vi "资讯打标签-打印函数 - 副本.vi"(6 "错误输入（无错误）":errorcluster caption="print error in", 7 "label num":i32, 8 "print path local":bool, 9 "PRINT":refnum<k24>, 10 "SN":refnum<k24>, 11 "SN输入":string="000019120-SD-R/Z00A2R1553S") -> (3 "printPath":string, 4 "print error":errorcluster caption="print error out")   [LabVIEW 2011]
uses:
  Data/ClassLibraryMisWebservice.dll
panel:
  out "Temp":string
  out "strPrintContent":string
  out "PrintSFCFSNLabel":string="OK"
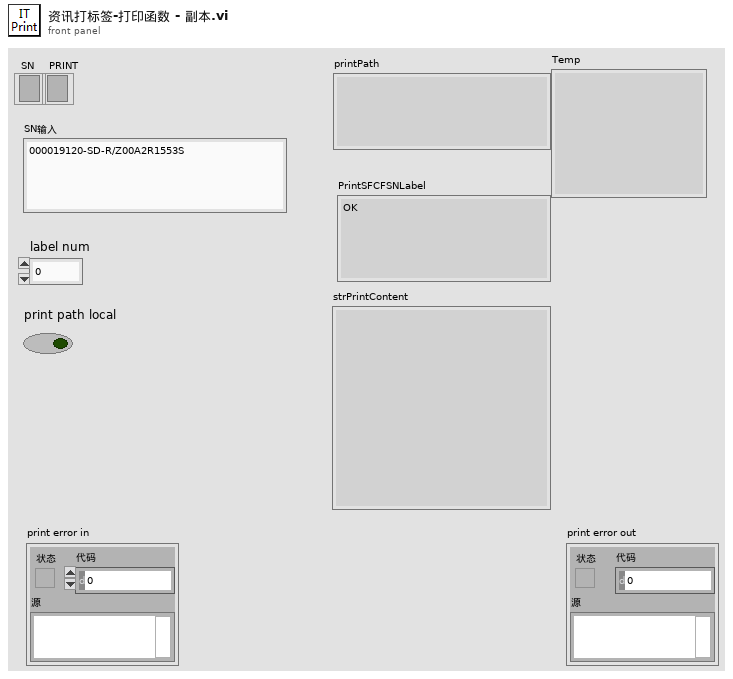
[diagram p1: front panel]
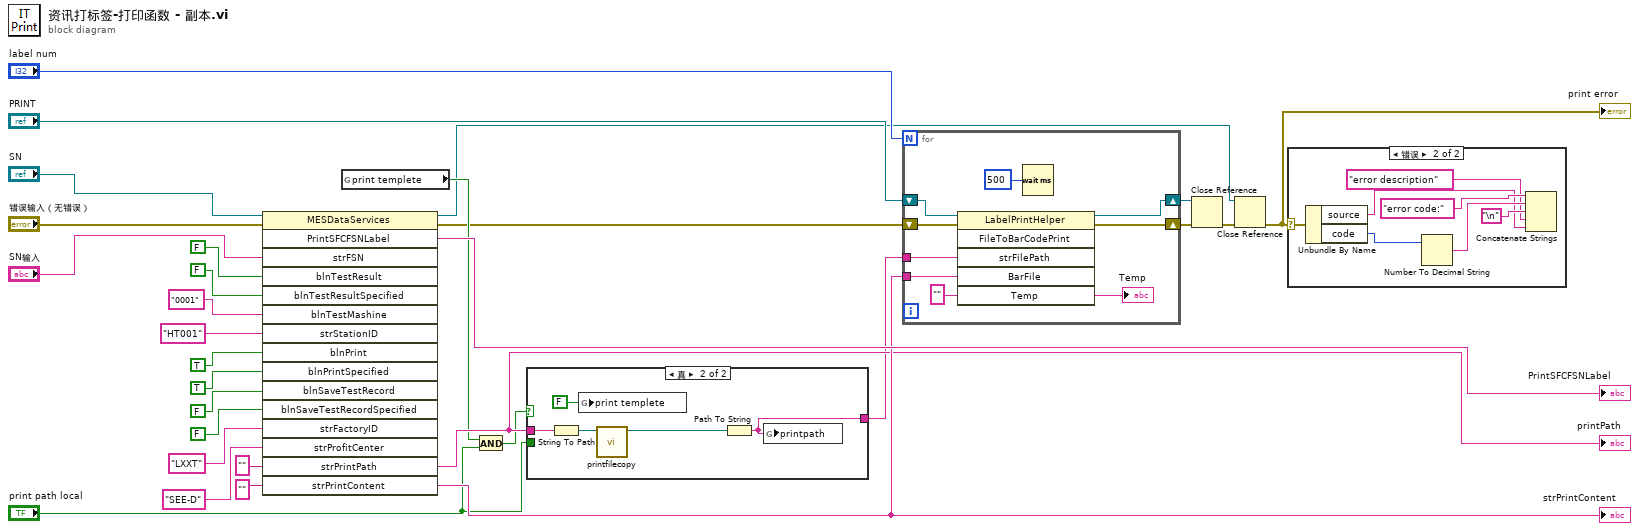
[diagram p0: block diagram]
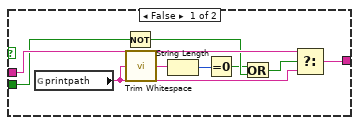
[diagram p3: hidden frame]
diagram:
  n1 = invoke class="MESDataServices" method="PrintSFCFSNLabel"(reference="SN", error in="错误输入（无错误）", "strFSN"="SN输入", "blnTestResult"=FALSE, "blnTestResultSpecified"=FALSE, "blnTestMashine"="0001", "strStationID"="HT001", "blnPrint"=TRUE, "blnPrintSpecified"=TRUE, "blnSaveTestRecord"=FALSE, "blnSaveTestRecordSpecified"=FALSE, "strFactoryID"="LXXT", "strProfitCenter"="SEE-D", "strPrintPath"="" ("printPath"), "strPrintContent"="") -> (reference out=w2:refnum<k24>, error out=w8:errorcluster, "PrintSFCFSNLabel"=→"PrintSFCFSNLabel":string, "strPrintPath"=w14:string, "strPrintContent"=w16:string)  [unwired: 1 in, 11 out]
  "printPath" <- w14
  "strPrintContent" <- w16
  n2 = global read "全局.vi" "print templete"() -> (w12:bool)
  n3 = And(x=w12, y="print path local") -> (x .and. y?=w11:bool)
  n4 = case shown="真" w11 {
    tunnel: w14 -> [w37 w44]
    tunnel: [w35 w40] -> w13
    tunnel: "print path local" -> [w34 _]
    frame False {
      n5 = global read "全局.vi" "printpath"() -> (w36:string)
      n6 = Not(x=w34) -> (.not. x?=w33:bool)
      n7 = call <vilib>:"Trim Whitespace.vi"("string"=w36) -> ("trimmed string"=w39:string)  [unwired: 1 in]
      n8 = String Length(string=w39) -> (length=w38:i32)
      n9 = Equal To 0?(x=w38) -> (x = 0?=w32:bool)
      n10 = Or(x=w32, y=w33) -> (x .or. y?=w31:bool)
      n11 = Select(t=w37, s=w31, f=w36) -> (s? t:f=w35:string)
    }
    frame True {
      n12 = String To Path(string=w44) -> (path=w43:path)
      n13 = global write "全局.vi" "print templete"(FALSE ("print templete")) -> ()
      n14 = call "printfilecopy.vi"("源路径"=w43) -> ("new path"=w42:path)  [unwired: 9 in, 1 out]
      n15 = Path To String(path=w42) -> (string=w40:string)
      n16 = global write "全局.vi" "printpath"(w40) -> ()
    }
  }
  n17 = for {
    N: "label num" -> [_]
    tunnel: w16 -> [w53]
    tunnel: w13 -> [w50]
    shift-right: [w47] -> w6
    shift-left: w8 -> [w48]
    shift-right: [w45] -> w4
    shift-left: "PRINT" -> [w46]
    n18 = invoke class="LabelPrintHelper" method="FileToBarCodePrint"(reference=w46, error in=w48, "strFilePath"=w50, "BarFile"=w53, "Temp"="") -> (reference out=w45:refnum<k24>, error out=w47:errorcluster, "Temp"=→"Temp":string)  [unwired: 1 in, 3 out]
    n19 = Wait (ms)(milliseconds to wait=u32 500 ("等待时间（毫秒）")) -> ()  [unwired: 1 out]
  }
  n20 = Close Reference(reference=w4, error in (no error)=w6) -> (error out=w3:errorcluster)
  n21 = Close Reference(reference=w2, error in (no error)=w3) -> (error out=w1:errorcluster)
  "print error" <- w1
  n22 = case shown="错误" w1 {
    selector: w1 -> [_ w60]
    frame No Error {
    }
    frame Error {
      n23 = Unbundle By Name(w60) -> ("source"=w55:string, "code"=w54:i32)
      n24 = Number To Decimal String(number=w54) -> (decimal integer string=w58:string)  [unwired: 1 in]
      n25 = Concatenate Strings("error code:" ("字符串"), w58, "\n", "error description" ("字符串"), w55) -> ()  [unwired: 1 out]
    }
  }
